vi "Find variables.vi"(11 "XML":string) -> (1 "Full Names":string[][](array[string]), 2 "Variable Clusters out":T1, 3 "Name":string[](array[string]))   [LabVIEW 2015, in "AguaClara Library.lvlib"]
uses:
  ADT 2/AguaClara Library.lvlib
  ADT 2/Variable cluster.ctl
panel:
  out "Name.Sub":string[](array[string])
  out "After Var Name":string[](array[string])
  in  "Variable Clusters":T1
  in  "regular expression":string="<ml:id xml:space=\"preserve\" subscript=\"[~\"<>]*\""
  # "check for unitoverride (a boolean)\n<ml:unitOverride>\n\nCheck for"
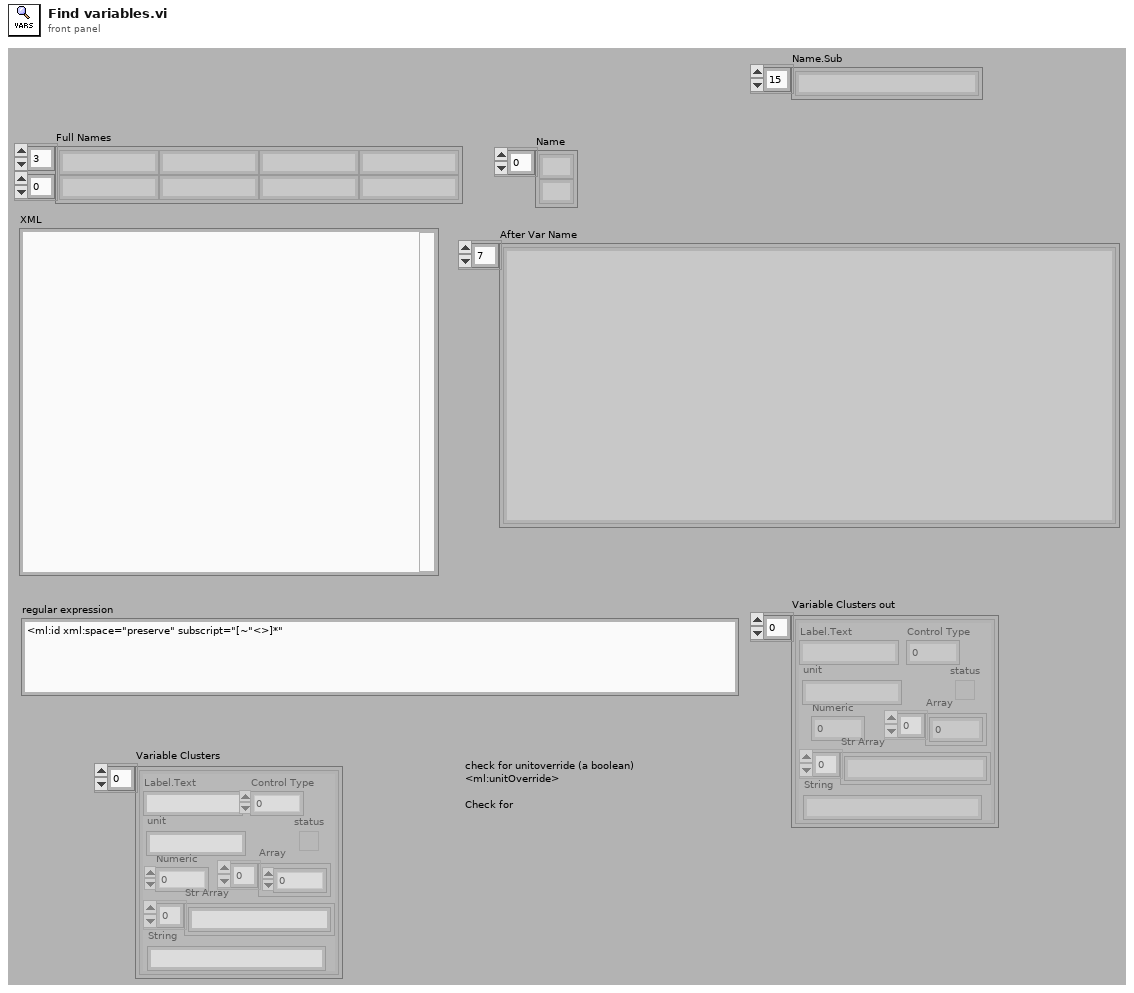
[diagram p1: front panel]
types:
  T1 = typedef "Variable cluster.ctl" = cluster{"Label.Text":string, "Control Type":u32, "Numeric":dbl, "Array":dbl[], "status":bool, "Str Array":string[], "String":string, "unit":string}[]
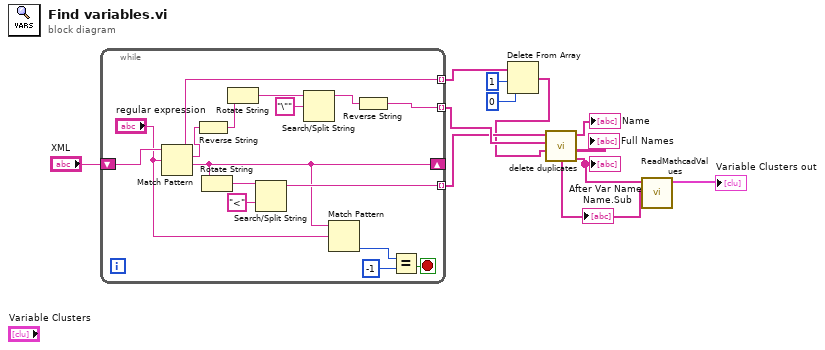
[diagram p0: block diagram]
diagram:
  n1 = while {
    shift-right: [w14] -> _
    shift-left: "XML" -> [w28]
    tunnel: [w25] -> w12 mode=indexing
    tunnel: [w18] -> w11 mode=indexing
    tunnel: [w16] -> w7 mode=indexing
    stop <- w27 stop-if-true
    n2 = Match Pattern(string=w28, regular expression="regular expression") -> (before substring=w16:string, match substring=w17:string, after substring=w14:string)  [unwired: 1 in, 1 out]
    n3 = Reverse String(1:w17) -> (0:w22:string)
    n4 = Rotate String(1:w14) -> (0:w20:string)
    n5 = Rotate String(1:w22) -> (0:w21:string)
    n6 = Search/Split String(string=w20, search string/char (-)="<") -> (substring before match=w18:string)  [unwired: 1 in, 2 out]
    n7 = Search/Split String(string=w21, search string/char (-)="\"") -> (substring before match=w23:string)  [unwired: 1 in, 2 out]
    n8 = Match Pattern(string=w14, regular expression="regular expression") -> (offset past match=w13:i32)  [unwired: 1 in, 3 out]
    n9 = Reverse String(1:w23) -> (0:w25:string)
    n10 = Equal?(x=w13, y=-1) -> (x = y?=w27:bool)
  }
  n11 = Delete From Array(array=w7, length=1, index=0) -> (array with subset deleted=w4:string[])  [unwired: 1 out]
  n12 = call "delete duplicates.vi"("After Var Name"=w4, "subscripts"=w12, "Name"=w11) -> ("After Var Name Out"=w3:string[], "Full Names"=→"Full Names":string[][], "Name Out"=→"Name":string[], "Name.Sub"=w2:string[])  [unwired: 4 in, 1 out]
  "After Var Name" <- w3
  "Name.Sub" <- w2
  n13 = call "ReadMathcadValues.vi"("Name.Sub"=w2, "After Var Name"=w3) -> ("Variable Clusters out"=→"Variable Clusters out":T1)  [unwired: 9 in]
